vi "Test Fails Generate Received Approved stays the same..vi"() -> ()   [LabVIEW 2020, in "Basic Mechanics Tests.lvclass"]
uses:
  Source/Approval Tests/Options/Options.lvclass
  Source/Approval Tests/Report Nothing/Report Nothing.lvclass
  C:/Users/SAS/Desktop/ApprovalTests.LabVIEW/Source/Approval Tests/Reporter/Reporter.lvclass
  Source/Approval Tests/Options/Options.lvclass/Options.ctl
  Source/Approval Tests/Naming Data/Naming Data.lvclass/Naming Data.ctl
  d27a92d8-1944-4452-9057-093efe2cb2fc.vi
  Source/Approval Tests/Options/Write Reporter.vi
  d27a92d8-1944-4452-9057-093efe2cb2fc.vi/93c5622b-9fb7-41e0-8c76-3fde37e94e34.vi
  Source/Approval Tests/Verify Core.vi
  Source/Approval Tests/Update Test Name if Not Defined.vi
  Source/Approval Tests/Options/Read Scrubber.vi
  d27a92d8-1944-4452-9057-093efe2cb2fc.vi/93c5622b-9fb7-41e0-8c76-3fde37e94e34.vi/04cb982b-2eda-40d0-8d7e-90f8e0b569b2.vi
  Source/Approval Tests/Options/Read Namer.vi
  Source/Approval Tests/Options/Read Naming Data.vi
  Source/Approval Tests/Options/Read Reporter.vi
  Source/Approval Tests/Naming Data/Read Test VI Name.vi
  Source/Approval Tests/Naming Data/Write Test VI Name.vi
  Source/Approval Tests/conv EOL.vi
  <vilib>/Utility/libraryn.llb/Check if File or Folder Exists.vi
  Source/Approval Tests/Reporter/Report.vi
  <vilib>/addons/_JKI Toolkits/Caraya/classes/Assert/Assert False.vi
  <vilib>/addons/_JKI Toolkits/Caraya/classes/Assert/Assert Equal Value_Variant.vi
  Source/Approval Tests/Scrubber/Scrubber.lvclass
  Source/Approval Tests/Namer/Namer.lvclass
  Source/Approval Tests/Naming Data/Naming Data.lvclass
  Source/Approval Tests/Reporter/Reporter.lvclass
  Basic Mechanics Tests.lvclass
  Basic Mechanics Tests.lvclass/Basic Mechanics Tests.ctl
  <vilib>/addons/_JKI Toolkits/Caraya/classes/Test/Test.lvclass
  <vilib>/addons/_JKI Toolkits/Caraya/classes/Assert/Assert.lvclass
  C:/Users/SAS/Desktop/ApprovalTests.LabVIEW/Source/Approval Tests/Report Nothing/Report Nothing.lvclass
panel:
  out "error out":errorcluster
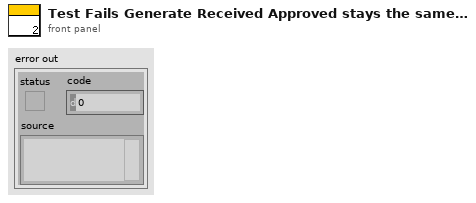
[diagram p1: front panel]
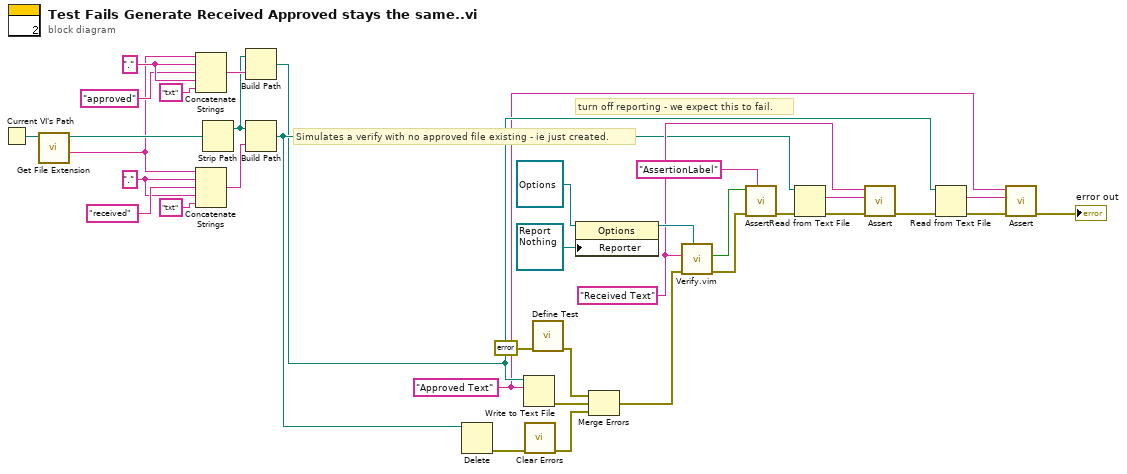
[diagram p0: block diagram]
diagram:
  w1 = "Approved Text"
  w22 = "." ("string")
  w27 = "." ("string")
  w16 = "Received Text"
  # "turn off reporting - we expect this to fail."
  # "Simulates a verify with no approved file existing - ie just created."
  n1 = Current VI's Path() -> (path=w29:path)
  n2 = call <vilib>:"Get File Extension.vi"("file"=w29) -> ("filename without extension"=w21:string, "dup file"=w28:path)  [unwired: 6 in, 3 out]
  n3 = Concatenate Strings(w21, w27, "approved" ("string"), w27, "txt" ("string")) -> (w25:string)
  n4 = Concatenate Strings(w21, w22, "received" ("string"), w22, "txt" ("string")) -> (w24:string)
  n5 = Strip Path(path=w28) -> (stripped path=w12:path)  [unwired: 1 out]
  n6 = Build Path(base path=w12, name or relative path=w25) -> (appended path=w2:path)
  n7 = Build Path(base path=w12, name or relative path=w24) -> (appended path=w3:path)
  n8 = Delete(path (use dialog)=w3) -> (error out=w9:errorcluster)  [unwired: 4 in, 2 out]
  n9 = Write to Text File(file (use dialog)=w2, text=w1) -> (error out=w8:errorcluster)  [unwired: 2 in, 2 out]
  n10 = call <vilib>:"Clear Errors.vi"("error in (no error)"=w9) -> ("error out"=w7:errorcluster)  [unwired: 5 in, 1 out]
  n11 = call <vilib>:"Define Test.vi"("error in (no error)"=errorcluster {"status"=FALSE, "code"=0, "source"=""}) -> ("error out"=w4:errorcluster)  [unwired: 9 in, 1 out]
  n12 = property on="Property Node" class="Options"(reference=refnum<class "Options.lvclass"> refnum ("Options"), "Reporter"=refnum<class "Report Nothing.lvclass"> refnum ("Approval Tests.lvlib:Report Nothing")) -> (reference out=w34:refnum<class "Options.lvclass">)  [unwired: 1 in, 1 out]
  n13 = Merge Errors(w4, w8, w7) -> (w6:errorcluster)
  n14 = call "Verify.vim"("Options"=w34, "error in"=w6, "Anything"=w16) -> ("error out"=w5:errorcluster, "Passed?"=w30:bool)  [unwired: 6 in, 1 out]
  n15 = call-poly <vilib>:"Assert.vi"("Label"="AssertionLabel" ("Label (VI Title)"), "error in (no error)"=w5, "False?"=w30) -> ("error out"=w20:errorcluster)  [unwired: 7 in, 1 out]
  n16 = Read from Text File(file (use dialog)=w3, error in=w20) -> (text=w17:string, error out=w19:errorcluster)  [unwired: 2 in, 2 out]
  n17 = call-poly <vilib>:"Assert.vi"("error in (no error)"=w19, "Y"=w17, "X"=w16) -> ("error out"=w18:errorcluster)  [unwired: 7 in, 1 out]
  n18 = Read from Text File(file (use dialog)=w2, error in=w18) -> (text=w14:string, error out=w15:errorcluster)  [unwired: 2 in, 2 out]
  n19 = call-poly <vilib>:"Assert.vi"("error in (no error)"=w15, "Y"=w14, "X"=w1) -> ("error out"=→"error out":errorcluster)  [unwired: 7 in, 1 out]
